vi "Wait until Done.vi"(8 "error in (no error)":errorcluster, 10 "timeout [s]":dbl=-1.0, 11 "DSP in":refnum<class "DSP.lvclass">) -> (0 "error out":errorcluster, 3 "DSP out":refnum<class "DSP.lvclass">)   [LabVIEW 2009, in "MicroDAQ.lvlib" / "DSP.lvclass"]
uses:
  <instrlib>/MicroDAQ/Channel/DSP/DSP.lvclass
  <instrlib>/MicroDAQ/Mlink library wraper/mlink.lvlib
  <instrlib>/MicroDAQ/Channel/Channel.lvclass
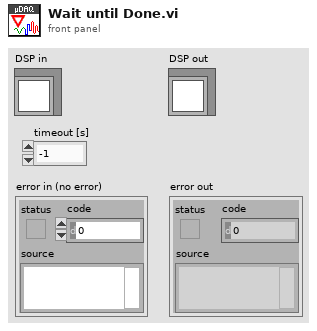
[diagram p1: front panel]
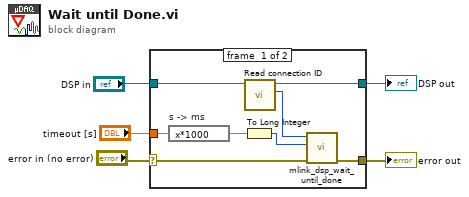
[diagram p0: block diagram]
diagram:
  n1 = case shown="No Error" "error in (no error)" {
    selector: "error in (no error)" -> [w13 w14]
    tunnel: [w12 w14] -> w4
    tunnel: "DSP in" -> [w11 w15]
    tunnel: [w10 w15] -> w2
    tunnel: "timeout [s]" -> [w6 _]
    frame #0 {
      n2 = expression code="x*1000" "s -> ms"(w6) -> (w8:dbl)
      n3 = To Long Integer(number=w8) -> (32bit integer=w7:i32)
      n4 = call <instrlib>:"Read connection ID.vi"("Task in"=w11) -> ("connection ID"=w9:i32, "Task out"=w10:refnum<class "DSP.lvclass">)  [unwired: 9 in]
      n5 = call <instrlib>:"mlink_dsp_wait_until_done.vi"("error in (no error)"=w13, "timeout"=w7, "connection ID"=w9) -> ("error out"=w12:errorcluster)  [unwired: 7 in, 1 out]
    }
    frame #1 {
    }
  }
  "error out" <- w4
  "DSP out" <- w2
